vi "NML VISA Open.vi"(7 "VISA Open timeout (0)":u32, 8 "error in (no error)":errorcluster, 9 "Access Mode":T1 items=["VISA Defaults"=0, "Exclusive Lock"=1, "Load Configured Settings"=4], 10 "duplicate session (T)":bool=TRUE, 11 "VISA resource name":refnum<visa-resource-name>) -> (0 "error out":errorcluster, 3 "VISA resource name out":refnum<visa-resource-name>)   [LabVIEW 2019]
uses:
  <vilib>/Instr/_visa.llb/VISA Open Access Mode.ctl
  Sub Controls/VISA Session Status.ctl
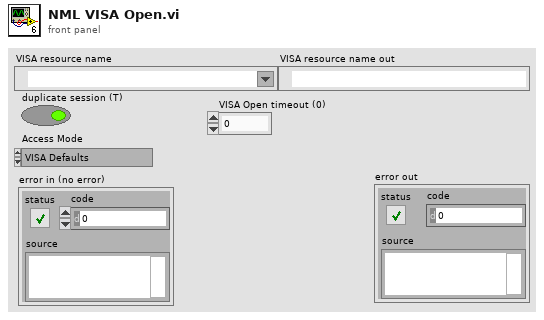
[diagram p1: front panel]
types:
  T1 = typedef "VISA Open Access Mode.ctl" = u32
  T2 = typedef "VISA Session Status.ctl" = enum16{"VISA Session Closed", "VISA Session Open", "VISA Session Locked"}
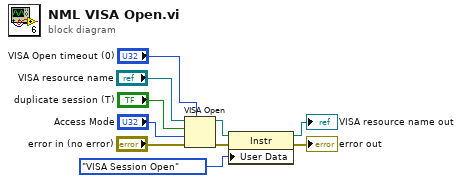
[diagram p0: block diagram]
diagram:
  n1 = VISA Open(timeout (0)="VISA Open timeout (0)", duplicate session (F)="duplicate session (T)", access mode="Access Mode", error in (no error)="error in (no error)", VISA resource name="VISA resource name") -> (VISA resource name=w4:refnum<visa-resource-name>, error out=w3:errorcluster)
  n2 = property class="Instr"(reference=w4, error in=w3, "User Data"=VISA_Session_Status."VISA Session Open") -> (reference out=→"VISA resource name out":refnum<visa-resource-name>, error out=→"error out":errorcluster)
